vi "switch_filter.vi"(2 "error in (no error)":errorcluster, 3 "VISA Refnum in":refnum<visa-resource-name>="COM4", 4 "fs":u32) -> (0 "error out":errorcluster, 1 "VISA Refnum out":refnum<visa-resource-name>)   [LabVIEW 2014]
panel:
  out "switch":u8
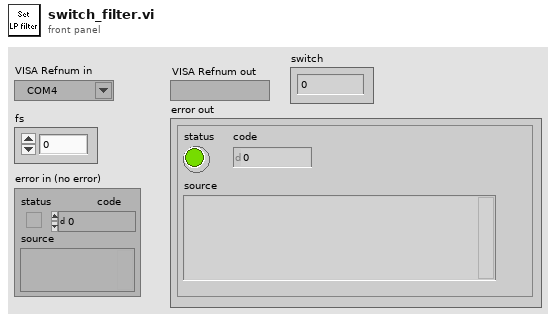
[diagram p1: front panel]
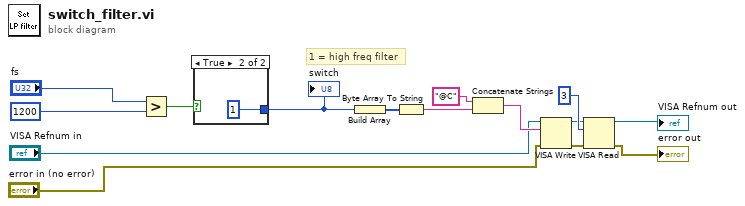
[diagram p0: block diagram]
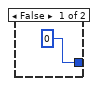
[diagram p2: hidden frame]
diagram:
  # "1 = high freq filter"
  n1 = Greater?(x="fs", y=u32 1200) -> (0:w15:bool)
  n2 = case shown="True" w15 {
    tunnel: [u8 0 u8 1] -> w14
    frame False {
    }
    frame True {
    }
  }
  "switch" <- w14
  n3 = Build Array(w14) -> (w8:u8[])
  n4 = Byte Array To String(unsigned byte array=w8) -> (string=w7:string)
  n5 = Concatenate Strings("@C" ("write buffer"), w7) -> (w12:string)
  n6 = VISA Write(VISA resource name="VISA Refnum in", write buffer=w12, error in (no error)="error in (no error)") -> (VISA resource name out=w10:refnum<visa-resource-name>, error out=w9:errorcluster)  [unwired: 1 out]
  n7 = VISA Read(VISA resource name=w10, byte count=u32 3, error in (no error)=w9) -> (VISA resource name out=→"VISA Refnum out":refnum<visa-resource-name>, error out=→"error out":errorcluster)  [unwired: 2 out]
